vi "TestConnection.vi"() -> ()   [LabVIEW 2014]
uses:
  <vilib>/Instr/_visa.llb/VISA Configure Serial Port (Instr).vi
panel:
  out "return count":u32
  out "State?":string
  out "Buffer Size":string
  out "CURR?":string
  out "Channel_state_a":string
  out "Channel_state_b":string
  in  "Keithley":refnum<visa-resource-name>
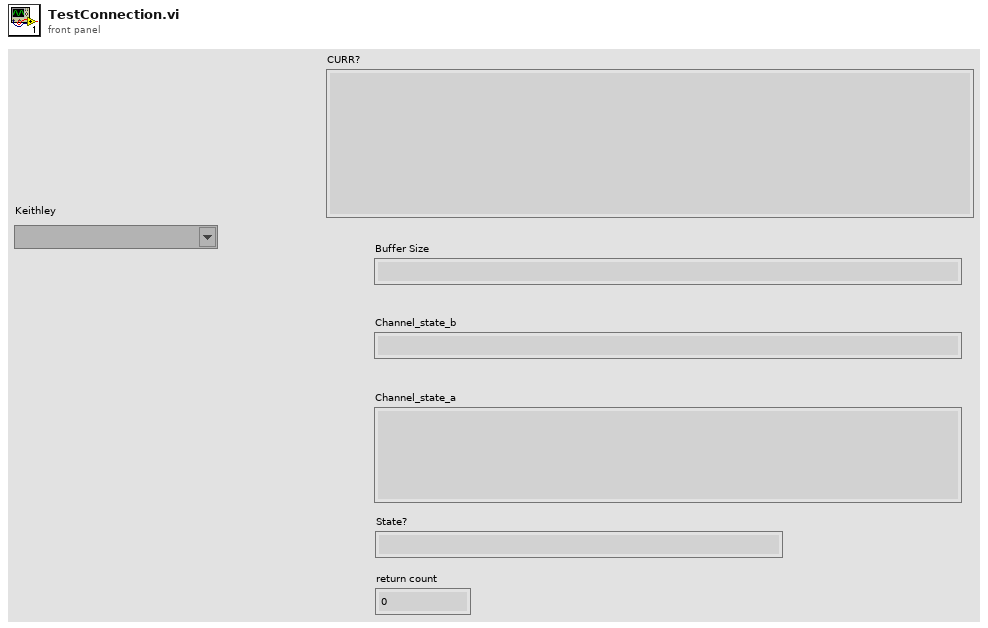
[diagram p1: front panel]
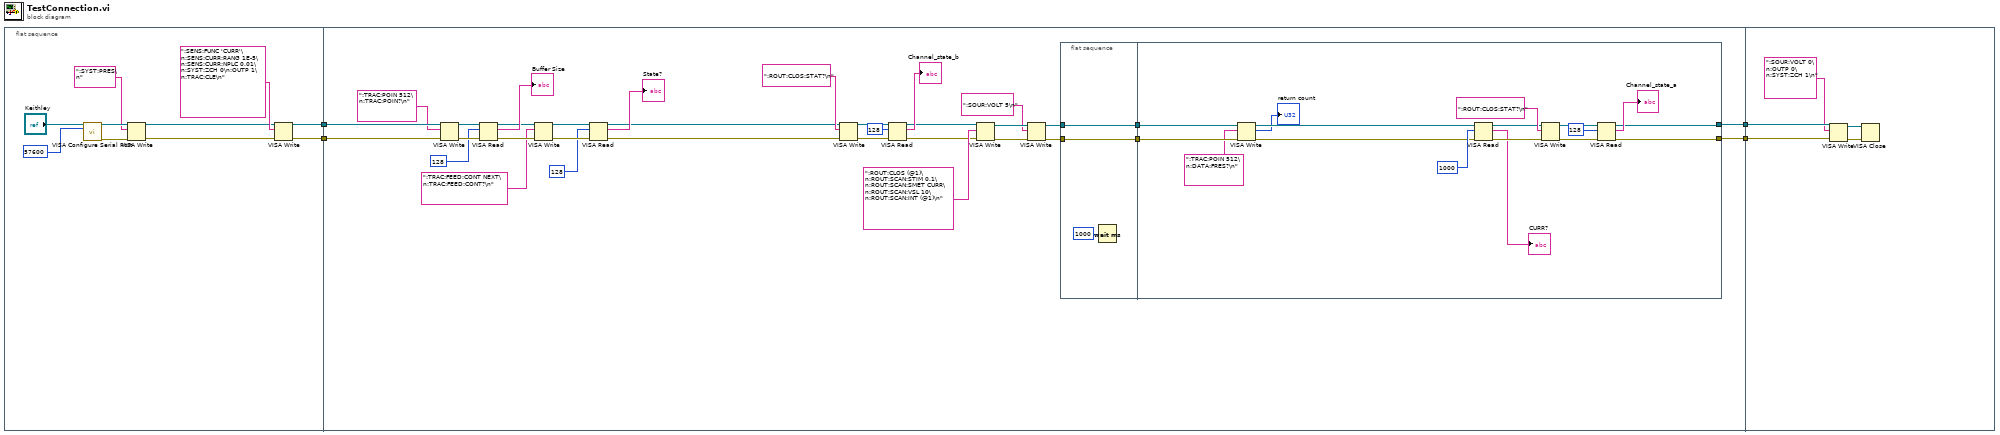
[diagram p0: block diagram]
diagram:
  n1 = flat-sequence {
    tunnel: [w6] -> w4
    tunnel: [w5] -> w3
    tunnel: w4 -> [w30]
    tunnel: w3 -> [w29]
    tunnel: [w41] -> w2
    tunnel: [w40] -> w1
    tunnel: w2 -> [w70]
    tunnel: w1 -> [w69]
    frame #0 {
      n2 = call-poly "VISA Configure Serial Port"("VISA resource name"="Keithley", "baud rate (9600)"=u32 57600) -> ("VISA resource name out"=w11:refnum<visa-resource-name>, "error out"=w10:errorcluster)  [unwired: 12 in]
      n3 = VISA Write(VISA resource name=w11, write buffer=":SYST:PRES\n", error in (no error)=w10) -> (VISA resource name out=w9:refnum<visa-resource-name>, error out=w8:errorcluster)  [unwired: 1 out]
      n4 = VISA Write(VISA resource name=w9, write buffer=":SENS:FUNC 'CURR'\n:SENS:CURR:RANG 1E-5\n:SENS:CURR:NPLC 0.01\n:SYST:ZCH 0\n:OUTP 1\n:TRAC:CLE\n", error in (no error)=w8) -> (VISA resource name out=w6:refnum<visa-resource-name>, error out=w5:errorcluster)  [unwired: 1 out]
    }
    frame #1 {
      n5 = VISA Write(VISA resource name=w30, write buffer=":TRAC:POIN 512\n:TRAC:POIN?\n", error in (no error)=w29) -> (VISA resource name out=w27:refnum<visa-resource-name>, error out=w26:errorcluster)  [unwired: 1 out]
      n6 = VISA Read(VISA resource name=w27, byte count=u32 128, error in (no error)=w26) -> (VISA resource name out=w23:refnum<visa-resource-name>, read buffer=→"Buffer Size":string, error out=w22:errorcluster)  [unwired: 1 out]
      n7 = VISA Write(VISA resource name=w23, write buffer=":TRAC:FEED:CONT NEXT\n:TRAC:FEED:CONT?\n", error in (no error)=w22) -> (VISA resource name out=w20:refnum<visa-resource-name>, error out=w19:errorcluster)  [unwired: 1 out]
      n8 = VISA Read(VISA resource name=w20, byte count=u32 128, error in (no error)=w19) -> (VISA resource name out=w16:refnum<visa-resource-name>, read buffer=→"State?":string, error out=w15:errorcluster)  [unwired: 1 out]
      n9 = VISA Write(VISA resource name=w16, write buffer=":ROUT:CLOS:STAT?\n", error in (no error)=w15) -> (VISA resource name out=w46:refnum<visa-resource-name>, error out=w45:errorcluster)  [unwired: 1 out]
      n10 = VISA Read(VISA resource name=w46, byte count=u32 128, error in (no error)=w45) -> (VISA resource name out=w39:refnum<visa-resource-name>, read buffer=→"Channel_state_b":string, error out=w38:errorcluster)  [unwired: 1 out]
      n11 = VISA Write(VISA resource name=w39, write buffer=":ROUT:CLOS (@1)\n:ROUT:SCAN:STIM 0.1\n:ROUT:SCAN:SMET CURR\n:ROUT:SCAN:VSL 10\n:ROUT:SCAN:INT (@1)\n", error in (no error)=w38) -> (VISA resource name out=w37:refnum<visa-resource-name>, error out=w36:errorcluster)  [unwired: 1 out]
      n12 = VISA Write(VISA resource name=w37, write buffer=":SOUR:VOLT 5\n", error in (no error)=w36) -> (VISA resource name out=w34:refnum<visa-resource-name>, error out=w33:errorcluster)  [unwired: 1 out]
      n13 = flat-sequence {
        tunnel: w33 -> [w49]
        tunnel: w34 -> [w50]
        tunnel: [w50] -> w32
        tunnel: [w49] -> w31
        tunnel: [w52] -> w41
        tunnel: [w51] -> w40
        tunnel: w32 -> [w59]
        tunnel: w31 -> [w58]
        frame #0 {
          n14 = Wait (ms)(milliseconds to wait=u32 1000) -> ()  [unwired: 1 out]
        }
        frame #1 {
          n15 = VISA Write(VISA resource name=w59, write buffer=":TRAC:POIN 512\n:DATA:FRES?\n", error in (no error)=w58) -> (VISA resource name out=w56:refnum<visa-resource-name>, return count=→"return count":u32, error out=w55:errorcluster)
          n16 = VISA Read(VISA resource name=w56, byte count=u32 1000, error in (no error)=w55) -> (VISA resource name out=w62:refnum<visa-resource-name>, read buffer=→"CURR?":string, error out=w61:errorcluster)  [unwired: 1 out]
          n17 = VISA Write(VISA resource name=w62, write buffer=":ROUT:CLOS:STAT?\n", error in (no error)=w61) -> (VISA resource name out=w65:refnum<visa-resource-name>, error out=w66:errorcluster)  [unwired: 1 out]
          n18 = VISA Read(VISA resource name=w65, byte count=u32 128, error in (no error)=w66) -> (VISA resource name out=w52:refnum<visa-resource-name>, read buffer=→"Channel_state_a":string, error out=w51:errorcluster)  [unwired: 1 out]
        }
      }
    }
    frame #2 {
      n19 = VISA Write(VISA resource name=w70, write buffer=":SOUR:VOLT 0\n:OUTP 0\n:SYST:ZCH 1\n", error in (no error)=w69) -> (VISA resource name out=w71:refnum<visa-resource-name>, error out=w72:errorcluster)  [unwired: 1 out]
      n20 = VISA Close(VISA resource name=w71, error in (no error)=w72) -> ()  [unwired: 1 out]
    }
  }
